vi "INA219 Code2Config.vi"(11 "Config Code":u16=15391 format="%04x") -> (3 "INA219 Config Options":T1={"Reset bit"=0, "Bus Voltage Range"=1, "PGA/Shunt Voltage Gain"=3, "Bus Voltage ADC Settings"=8, "Shunt Voltage ADC Settings"=3, "Mode"=7, "Calibration Value"=4096} {"Calibration Value" format="%.0x"; "Mode" items=["Power Down", "Shunt Voltage, Triggered", "Bus Voltage, Triggered", "Shunt & Bus, Triggered", "ADC Off (Disabled)", "Shunt Voltage, Continuous", "Bus Voltage, Continuous", "Shunt & Bus Voltage, Continuous"]; "Shunt Voltage ADC Settings" items=["9-bit, 84us conversion time"=0, "10-bit, 148us conversion time"=1, "11-bit, 276us conversion time"=2, "12-bit, 532us conversion time"=3, "1x12-bit, 532us conversion time"=8, "2x12-bit averaged, 1.06ms conversion time"=9, "4x12-bit averaged, 2.13ms conversion time"=10, "8x12-bit averaged, 4.26ms conversion time"=11, "16x12-bit averaged, 8.51ms conversion time"=12, "32x12-bit averaged, 17.02ms conversion time"=13, "64x12-bit averaged, 34.05ms conversion time"=14, "128x12-bit averaged, 68.10ms conversion time"=15]; "Bus Voltage ADC Settings" items=["9-bit, 84us conversion time"=0, "10-bit, 148us conversion time"=1, "11-bit, 276us conversion time"=2, "12-bit, 532us conversion time"=3, "1x12-bit, 532us conversion time"=8, "2x12-bit averaged, 1.06ms conversion time"=9, "4x12-bit averaged, 2.13ms conversion time"=10, "8x12-bit averaged, 4.26ms conversion time"=11, "16x12-bit averaged, 8.51ms conversion time"=12, "32x12-bit averaged, 17.02ms conversion time"=13, "64x12-bit averaged, 34.05ms conversion time"=14, "128x12-bit averaged, 68.10ms conversion time"=15]; "PGA/Shunt Voltage Gain" items=["Gain 1, +/-40mV", "Gain 2, +/-80mV", "Gain 3, +/-160mV", "Gain 4, +/-320mV"]; "Bus Voltage Range" items=["0-16V Range", "0-32V Range"]; "Reset bit" items=["Do Not Reset", "Reset"]})   [LabVIEW 2014]
uses:
  BMP180/BMP180 Config Options.ctl
panel:
  out "Config (binary)":bool[](array[boolean])
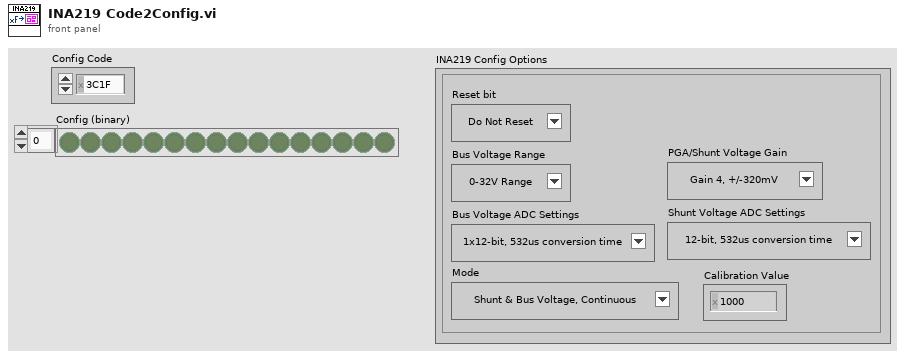
[diagram p1: front panel]
types:
  T1 = typedef "BMP180 Config Options.ctl" = cluster{"Reset bit":u8, "Bus Voltage Range":u8, "PGA/Shunt Voltage Gain":u8, "Bus Voltage ADC Settings":u8, "Shunt Voltage ADC Settings":u8, "Mode":u8, "Calibration Value":u16}
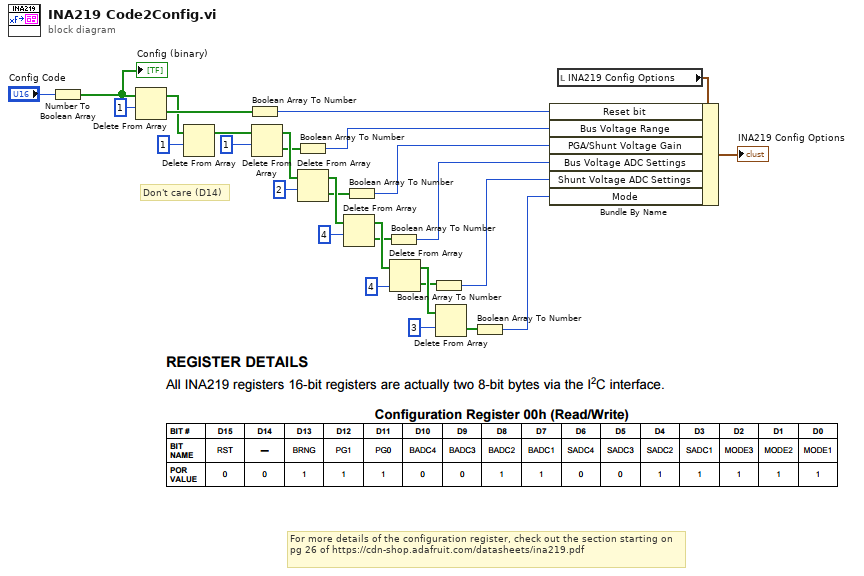
[diagram p0: block diagram]
diagram:
  # "Don't care (D14)"
  # "For more details of the configuration register, check out the section starting on pg 26 of https://cdn-shop.adafruit.com/datasheets/ina219.pdf"
  n1 = Number To Boolean Array(number="Config Code") -> (Boolean array=w26:bool[])
  "Config (binary)" <- w26
  n2 = Delete From Array(array=w26, length=1) -> (deleted portion=w24:bool[], array with subset deleted=w3:bool[])  [unwired: 1 in]
  n3 = Delete From Array(array=w3, length=1) -> (array with subset deleted=w2:bool[])  [unwired: 1 in, 1 out]
  n4 = Boolean Array To Number(Boolean array=w24) -> (number=w23:u32)
  n5 = Delete From Array(array=w2, length=1) -> (deleted portion=w12:bool[], array with subset deleted=w21:bool[])  [unwired: 1 in]
  n6 = Boolean Array To Number(Boolean array=w12) -> (number=w8:u32)
  n7 = Delete From Array(array=w21, length=2) -> (deleted portion=w13:bool[], array with subset deleted=w20:bool[])  [unwired: 1 in]
  n8 = Delete From Array(array=w20, length=4) -> (deleted portion=w11:bool[], array with subset deleted=w19:bool[])  [unwired: 1 in]
  n9 = Boolean Array To Number(Boolean array=w13) -> (number=w7:u32)
  n10 = Boolean Array To Number(Boolean array=w11) -> (number=w6:u32)
  n11 = Delete From Array(array=w19, length=4) -> (deleted portion=w10:bool[], array with subset deleted=w14:bool[])  [unwired: 1 in]
  n12 = Boolean Array To Number(Boolean array=w10) -> (number=w5:u32)
  n13 = Delete From Array(array=w14, length=3) -> (deleted portion=w9:bool[])  [unwired: 1 in, 1 out]
  n14 = Boolean Array To Number(Boolean array=w9) -> (number=w4:u32)
  n15 = local read "INA219 Config Options"() -> (w28:T1)
  n16 = Bundle By Name(cluster=w28, "Reset bit"=w23, "Bus Voltage Range"=w8, "PGA/Shunt Voltage Gain"=w7, "Bus Voltage ADC Settings"=w6, "Shunt Voltage ADC Settings"=w5, "Mode"=w4) -> (→"INA219 Config Options":T1)
